vi "Info Insert Row to 1D String Array.vi"(6 "source info data":string, 7 "key description":string, 8 "sections in":string[](array[string]), 9 "row index to insert":i32, 10 "string to insert":string, 11 "info data in":string) -> (0 "sections out":string[](array[string]), 3 "info data out":string)   [LabVIEW 2018]
doc: "Addition to infolib: Gets vertical 1D array of strings (if exits in the 'info data in'), inserts one string into it in selected row, writes it back."
uses:
  infolib.lvlibp/Private/Get matrix polymorph parts/Get 1D String.vi
  infolib.lvlibp/Private/Add matrix polymorph parts/1D String.vi
  infolib.lvlibp
panel:
  out "value":string[](array[string])
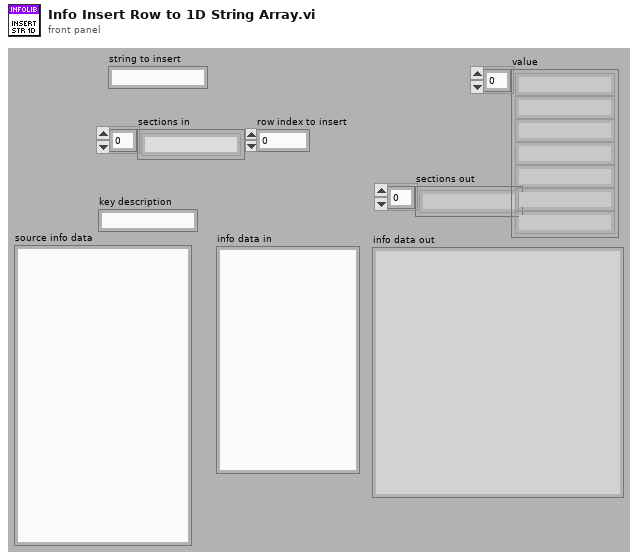
[diagram p1: front panel]
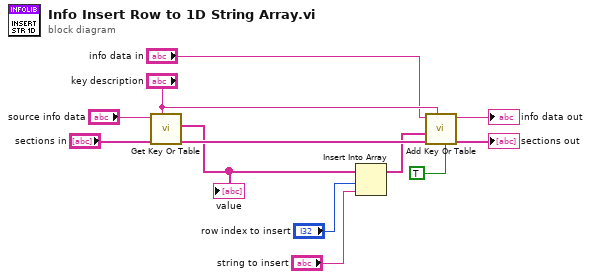
[diagram p0: block diagram]
diagram:
  n1 = call-poly "Get Key Or Table.vi"("key description"="key description", "sections"="sections in", "info data"="source info data") -> ("sections out"=w11:string[], "value"=w2:string[])  [unwired: 5 in, 2 out]
  "value" <- w2
  n2 = Insert Into Array(array=w2, index="row index to insert", new element="string to insert") -> (w5:string[])
  n3 = call-poly "Add Key Or Table.vi"("column vector (F)"=TRUE, "key description"="key description", "sections"=w11, "string"=w5, "info data"="info data in") -> ("sections out"=→"sections out":string[], "info data out"=→"info data out":string)  [unwired: 5 in]
